vi "Arduino RGB LED.vi"() -> ()   [LabVIEW 2011, in "LabVIEW Interface for Arduino.lvlib"]
doc: "An example that uses the Arduino's PWM pins to control an RGB LED."
uses:
  vi.lib/LabVIEW Interface for Arduino/LabVIEW Interface for Arduino.lvlib
panel:
  in  "VISA resource name":refnum<visa-resource-name>
  out "Color":u32(colorbox)
  in  "Blue":u8(slide) scale=0.0..255.0
  in  "Green":u8(slide) scale=0.0..255.0
  in  "Stop":bool
  in  "Red":u8(slide) scale=0.0..255.0
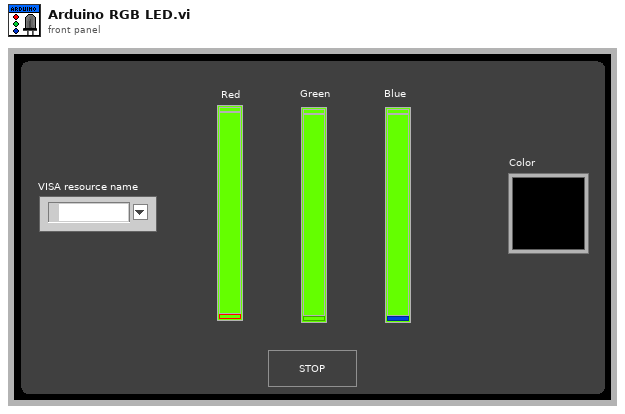
[diagram p1: front panel]
types:
  T1 = typedef "LabVIEW Interface for Arduino.lvlib/Arduino Resource.ctl" = cluster{"VISA resource":refnum<visa-resource-name>, "Board Type":T2, "Connection Type":enum8{"USB / Serial"}, "Bytes Per Packet (15)":u8}
  T2 = typedef "LabVIEW Interface for Arduino.lvlib/Board Type.ctl" = enum16{"Arduino Uno", "Dimuelanove w/Atmega 328", "Mega 2560", "Chipkit Uno32", "Chipkit Max32"}
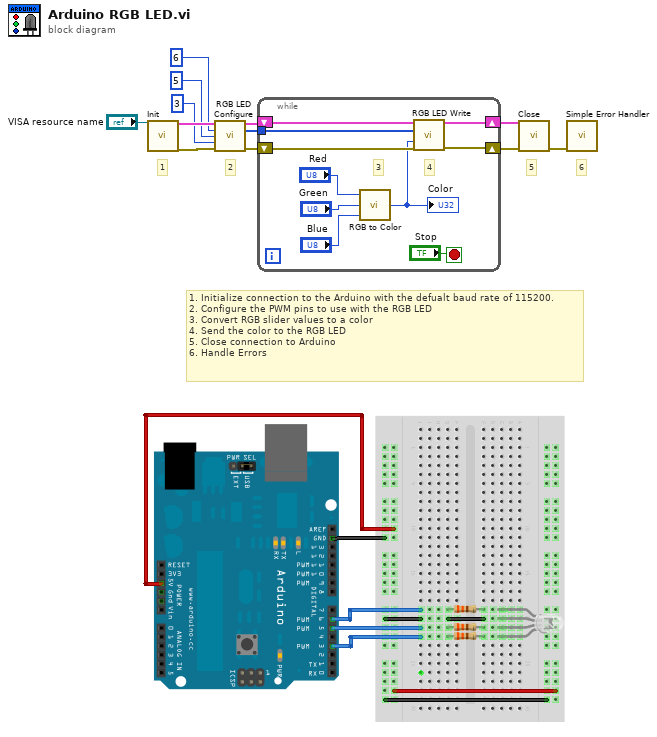
[diagram p0: block diagram]
diagram:
  # "6"
  # "5"
  # "2"
  # "1"
  # "1. Initialize connection to the Arduino with the defualt baud rate of 115200.\n2. Configure the PWM pins to use with the RGB LED\n3. Convert RGB slider values to a color\n4. Send the color to the RGB LED\n5. Close connection to Arduino\n6. Handle Errors"
  n1 = call "Init.vi"("VISA resource"="VISA resource name") -> ("Arduino Resource"=w10:T1, "error out"=w11:errorcluster)  [unwired: 17 in]
  n2 = call "RGB LED Configure.vi"("Arduino Resource"=w10, "Red Pin"=u8 6, "Green Pin"=u8 5, "Blue Pin"=u8 3, "error in"=w11) -> ("Arduino Resource"=w9:T1, "RGB LED Pins"=w2:u8[], "error out"=w8:errorcluster)  [unwired: 8 in]
  n3 = while {
    shift-right: [w22] -> w3
    shift-left: w9 -> [w14]
    shift-right: [w21] -> w12
    shift-left: w8 -> [w20]
    tunnel: w2 -> [w13]
    stop <- "Stop" stop-if-true
    # "4"
    # "3"
    n4 = call <vilib>:"RGB to Color.vi"("B"="Blue", "G"="Green", "R"="Red") -> ("Color"=w17:u32)
    "Color" <- w17
    n5 = call "RGB LED Write.vi"("Arduino Resource"=w14, "RGB LED Pins"=w13, "Color"=w17, "error in"=w20) -> ("Arduino Resource"=w22:T1, "error out"=w21:errorcluster)  [unwired: 9 in, 1 out]
  }
  n6 = call "Close.vi"("Arduino Resource"=w3, "error in"=w12) -> ("error out"=w7:errorcluster)  [unwired: 13 in]
  n7 = call <vilib>:"Simple Error Handler.vi"("error in (no error)"=w7) -> ()  [unwired: 4 in, 5 out]
